vi "保存波形文件.vi"() -> ()   [LabVIEW 2010]
uses:
  <vilib>/Waveform/WDTFileIO.llb/ Write Waveform to File.vi
  <vilib>/measure/NI_MABase.lvlib
panel:
  in  "文件路径":path=path "c:/file/w1"
  in  "采样参数":cluster{"采样率":dbl, "采样数":dbl}={"采样率"=1000.0, "采样数"=1000.0} {"采样数" format="%.2p"; "采样率" format="%.2p"}
  in  "幅值":dbl=1.0 format="%.2p"
  in  "频率":dbl=10.0 format="%.2p"
  out "波形图":waveform(dbl)(graph)
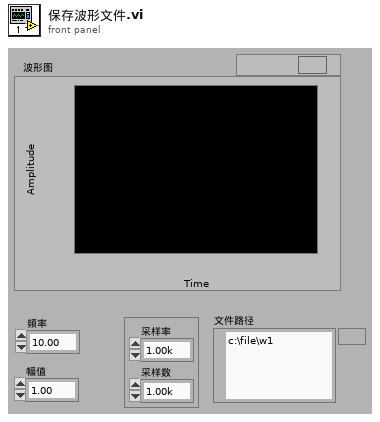
[diagram p1: front panel]
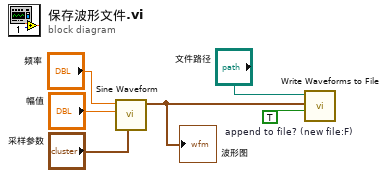
[diagram p0: block diagram]
diagram:
  w3 = TRUE  # append to file? (new file:F)
  n1 = call <vilib>:"Sine Waveform.vi"("sampling info"="采样参数", "amplitude"="幅值", "frequency"="频率") -> ("signal out"=w1:waveform(dbl))  [unwired: 7 in, 1 out]
  "波形图" <- w1
  n2 = call-poly <vilib>:"Write Waveforms to File.vi"("append to file? (new file:F)"=w3, "waveform"=w1, "file path (dialog if empty)"="文件路径") -> ()  [unwired: 7 in, 2 out]
